vi "SERIAL_DecodeAHRS.vi"() -> ()   [LabVIEW 2014, in "navX Library v1 (deprecated).lvlib"]
uses:
  navX Library v1 (deprecated).lvlib
panel:
  out "Valid?":bool
  in  "navX Data":u8[](array[numeric])
  out "navX Data":u8[](array[numeric])
  in  "Buffer":string
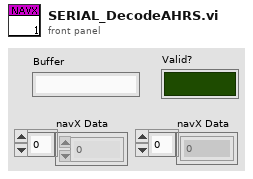
[diagram p1: front panel]
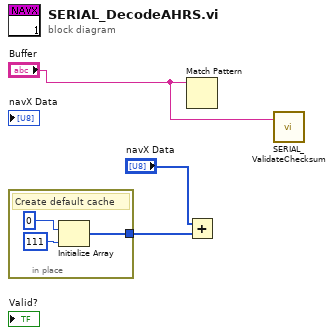
[diagram p0: block diagram]
diagram:
  n1 = in-place {
    in-place-border: [w4] -> w3
    # "Create default cache"
    n2 = Initialize Array(u8 0 ("Received Data"), u8 111 ("hex")) -> (w4:u8[])
  }
  n3 = Match Pattern(string="Buffer") -> ()  [unwired: 2 in, 4 out]
  n4 = Add(x="navX Data", y=w3) -> ()  [unwired: 1 out]
  n5 = call "SERIAL_ValidateChecksum.vi"("Content"="Buffer") -> ()  [unwired: 1 in, 1 out]
